vi "Limitador_Multiplicador.vi"(10 "IN":dbl) -> (2 "OUT":dbl)   [LabVIEW 2020]
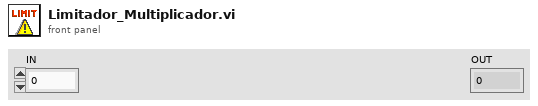
[diagram p1: front panel]
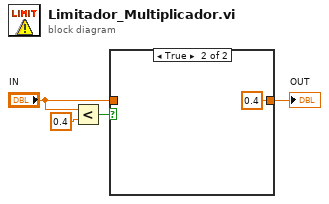
[diagram p0: block diagram]
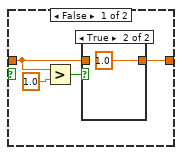
[diagram p2: hidden frame]
diagram:
  n1 = Less?(x="IN", y=0.4) -> (x < y?=w3:bool)
  n2 = case shown="True" w3 {
    tunnel: [w5 0.4] -> w2
    tunnel: "IN" -> [w6 _]
    frame False {
      n3 = Greater?(x=w6, y=1.0) -> (0:w8:bool)
      n4 = case shown="True" w8 {
        tunnel: w6 -> [w9 _]
        tunnel: [w9 1.0] -> w5
        frame False {
        }
        frame True {
        }
      }
    }
    frame True {
    }
  }
  "OUT" <- w2
